vi "Replace Aliases with Endpoints.vi"(10 "Alias Mappings":T2[](array[typedef]), 11 "UI Connections List in":T1[](array[typedef])) -> (3 "UI Connections List out":T1[](array[typedef]))   [LabVIEW 2020, in "Routing and Faulting System Explorer.lvlib"]
uses:
  Routing and Faulting System Explorer.lvlib
  Shared/Alias Mapping.ctl
  Shared/Alias Endpoint.ctl
  Connection Row.ctl
  Form Endpoint.vi
  Shared/Routing and Faulting Shared.lvlib
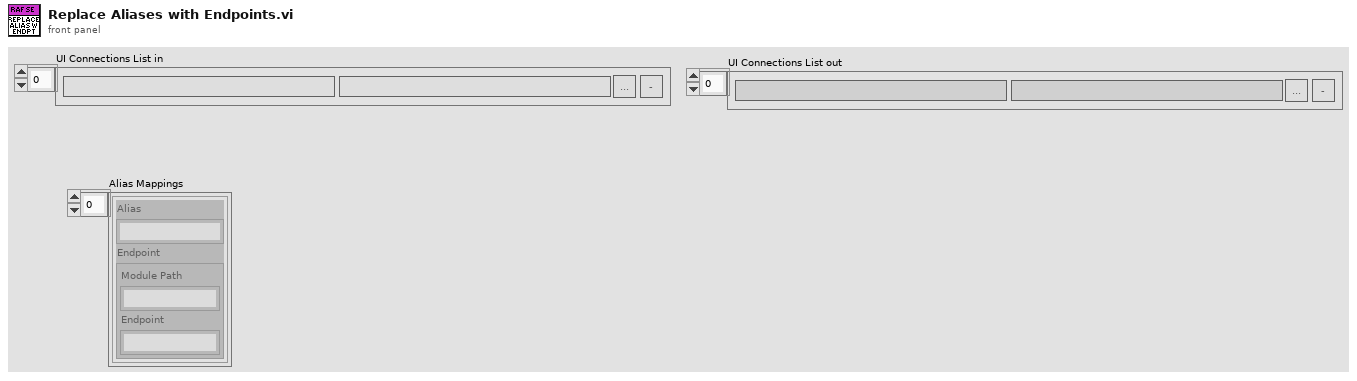
[diagram p1: front panel]
types:
  T1 = typedef "Routing and Faulting System Explorer.lvlib/Connection Row.ctl" = cluster{"Source":string, "Destination":string, "Edit":bool, "Remove":bool}
  T2 = typedef "Routing and Faulting Shared.lvlib/Alias Mapping.ctl" = cluster{"Alias":string, "Endpoint":T3}
  T3 = typedef "Routing and Faulting Shared.lvlib/Alias Endpoint.ctl" = cluster{"Module Path":string, "Endpoint":string}
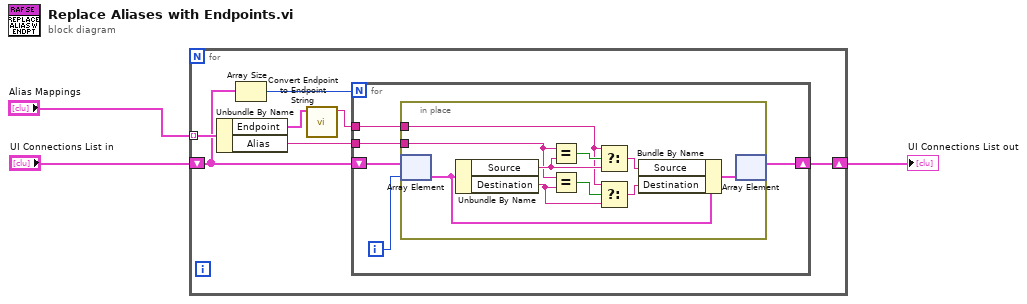
[diagram p0: block diagram]
diagram:
  n1 = for {
    tunnel: "Alias Mappings" -> [w10] mode=indexing
    shift-right: [w8] -> w2
    shift-left: "UI Connections List in" -> [w7]
    n2 = Unbundle By Name(w10) -> ("Endpoint"=w5:T3, "Alias"=w9:string)
    n3 = Array Size(array=w7) -> (size(s)=w6:i32)
    n4 = call "Convert Endpoint to Endpoint String.vi"("Endpoint"=w5) -> ("Endpoint String"=w4:string)  [unwired: 10 in]
    n5 = for {
      N: w6 -> [_]
      tunnel: w4 -> [w14]
      tunnel: w9 -> [w13]
      shift-right: [w12] -> w8
      shift-left: w7 -> [w15]
      i -> [w11]
      n6 = in-place {
        in-place-border: w14 -> [w17]
        in-place-border: w13 -> [w16]
        n7 = in-place-array #1(w15, w11) -> (w19:T1)
        n8 = Unbundle By Name(w19) -> ("Source"=w22:string, "Destination"=w24:string)
        n9 = Equal?(x=w16, y=w22) -> (x = y?=w20:bool)
        n10 = Equal?(x=w16, y=w24) -> (x = y?=w23:bool)
        n11 = Select(t=w17, s=w20, f=w22) -> (s? t:f=w21:string)
        n12 = Select(t=w17, s=w23, f=w24) -> (s? t:f=w25:string)
        n13 = Bundle By Name(cluster=w19, "Source"=w21, "Destination"=w25) -> (w18:T1)
        n14 = in-place-array #1(w18) -> (w12:T1[])  [unwired: 1 out]
      }
    }
  }
  "UI Connections List out" <- w2
